vi "Main.vi"() -> ()   [LabVIEW 2020]
uses:
  Def/MHL_Data.ctl
  Def/Queue_Function Def.ctl
  Def/Queue_Method Def.ctl
  Def/Saving Type.ctl
  Def/Watchdog_Data.ctl
  Def/Event Log.ctl
  Objects/Saving Function/Saving OO/Save as csv/Save as csv.lvclass
  D:/Projects/practice/QMH+Producer_consumer/QMH+Producer_consumer/Objects/Saving Function/Saving OO/Saving OO.lvclass
  Def/Queue_Def.ctl
  <userlib>/_MGI/Timing/MGI Wait/MGI Wait (U32).vi
  Objects/Saving Function/Saving OO/Save as txt/Save as txt.lvclass
  Objects/Saving Function/Saving OO/Saving OO.lvclass
panel:
  in  "Connect/Reconnect":bool
  in  "Power":bool
  in  "Decrease Amplitude":bool
  in  "Add Amplitude":bool
  in  "Decrease Frequence":bool
  in  "Increase Frequence":bool
  out "Waveform":dynamicdata(graph)
  in  "MHL Data":T1={"Offset"=0.0, "Frequency"=10.1, "Amplitude"=1.0}
  out "Ver.#":string
  out "error out":errorcluster
  in  "error in (no error)":errorcluster
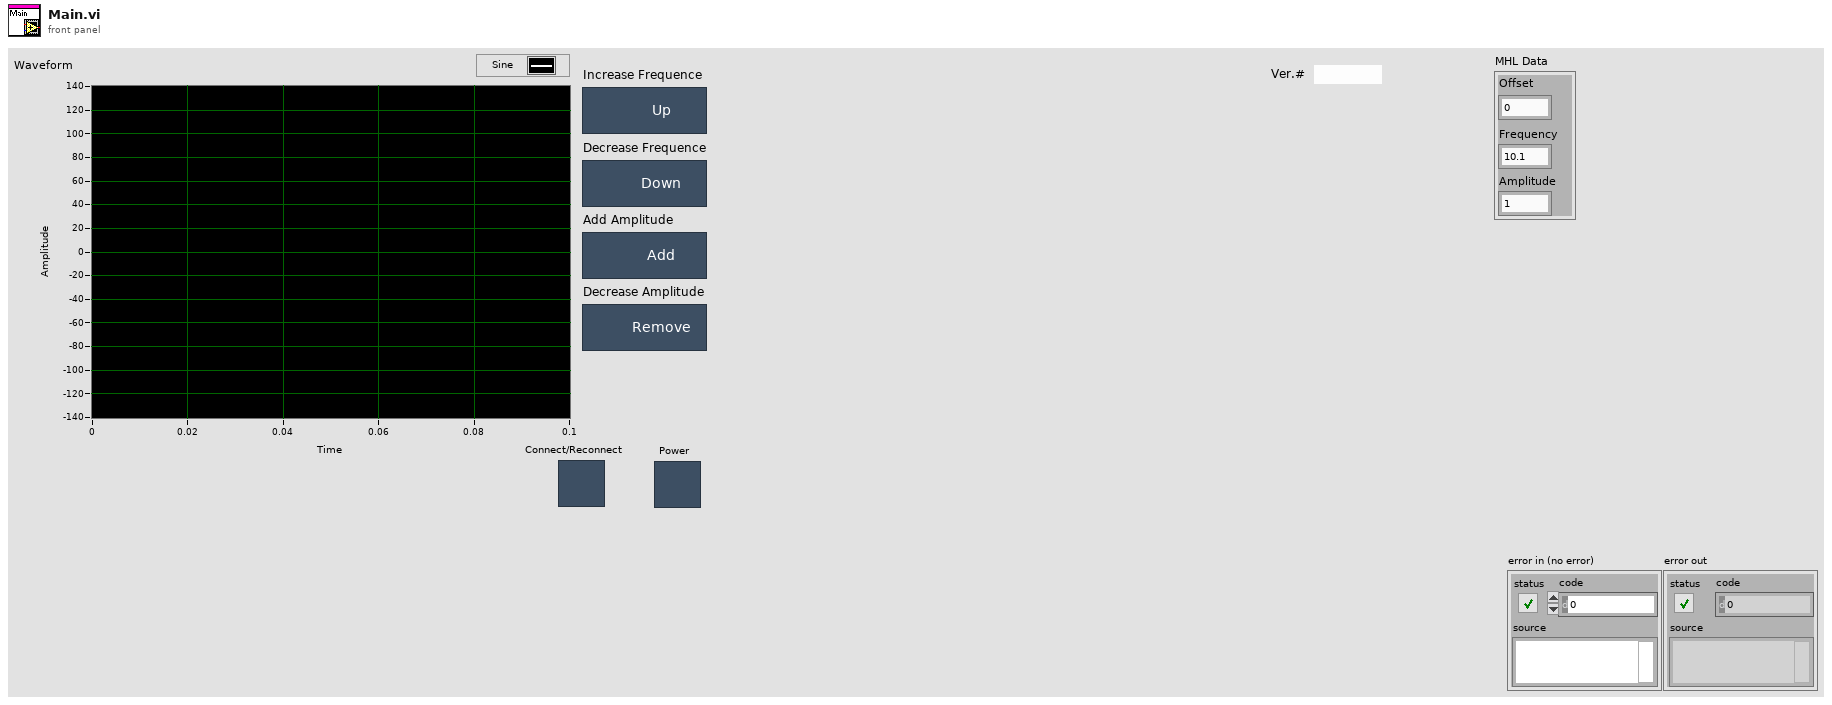
[diagram p1: front panel]
types:
  T1 = typedef "MHL_Data.ctl" = cluster{"Offset":dbl, "Frequency":dbl, "Amplitude":dbl}
  T2 = typedef "Event Log.ctl" = cluster{"Saving Path Folde":path}
  T3 = typedef "Watchdog_Data.ctl" = cluster{string}
  T4 = typedef "Queue_Method Def.ctl" = enum16{"Initialize", "Read", "Write", "Insert", "Get_Specific_Quene_Status", "Flush Speciffic Quene", "Release All Quenes"}
  T5 = typedef "Queue_Function Def.ctl" = enum16{"MHL", "Return(Watch dog)", "Event Log", "Error Log"}
  T6 = typedef "Saving Type.ctl" = enum16{"Default", "txt", "csv"}
  T7 = typedef "Main_Data_Package.ctl" = cluster{"This Vi Ref Out":refnum<vi>, "Map Out":map{string, refnum<vi>}, "User Event Out":refnum<user-event>, "User_Event Ref Reg":refnum<event-registration>, "Event Log Path":path}
  T8 = typedef "Queue_Def.ctl" = cluster{"Message":string, "Data":variant}
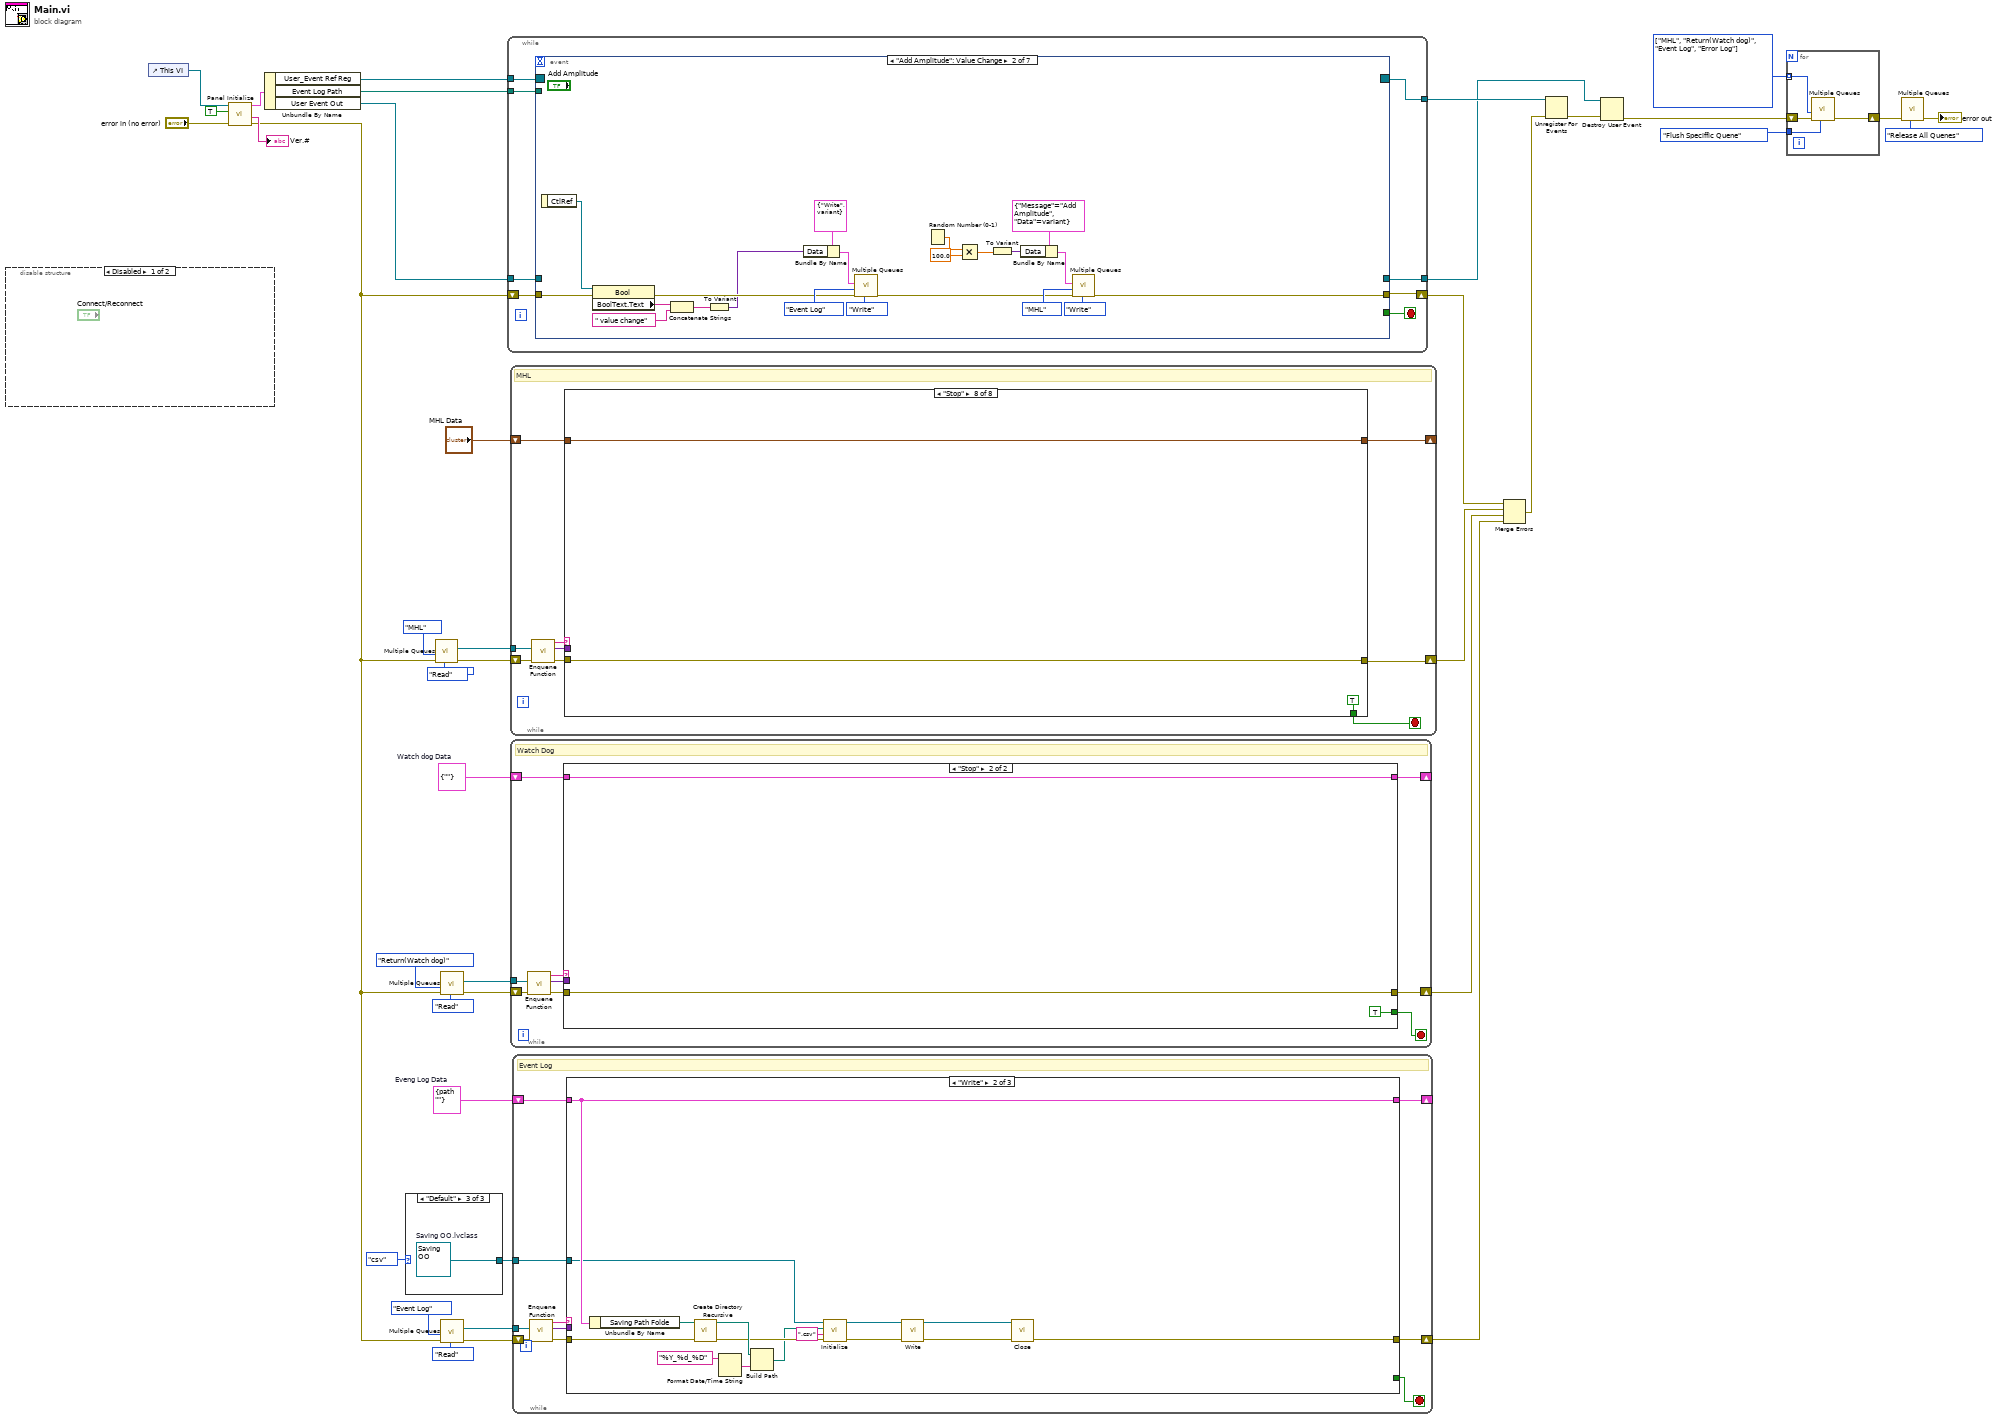
[diagram p0: block diagram]
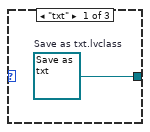
[diagram p3: hidden frame]
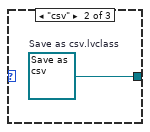
[diagram p4: hidden frame]
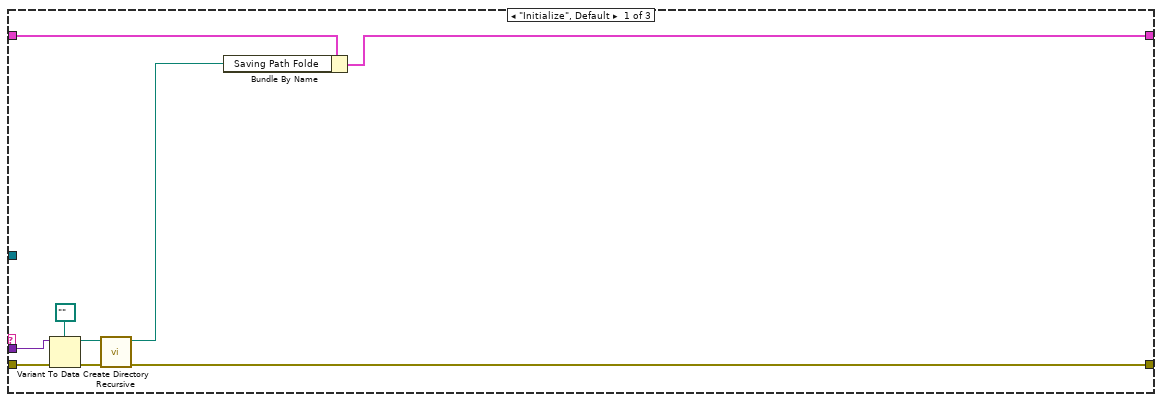
[diagram p5: hidden frame]
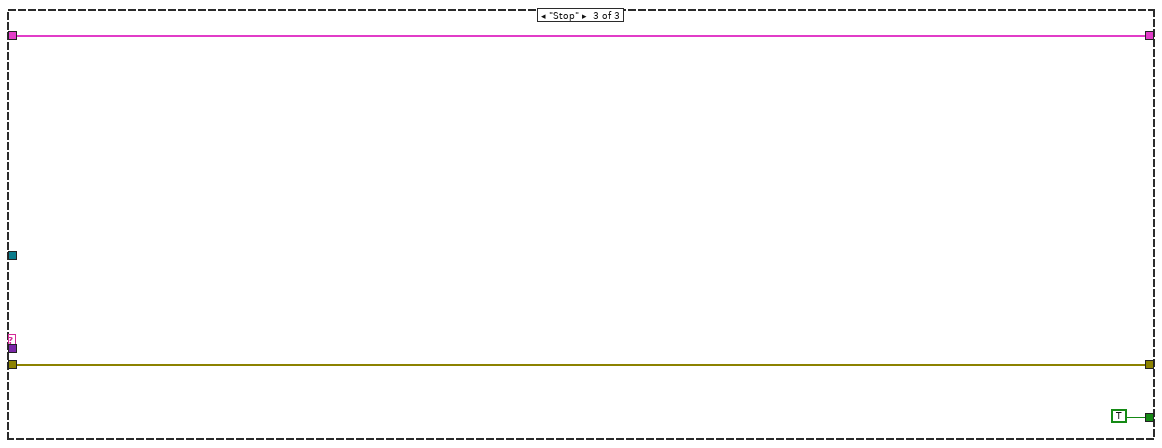
[diagram p6: hidden frame]
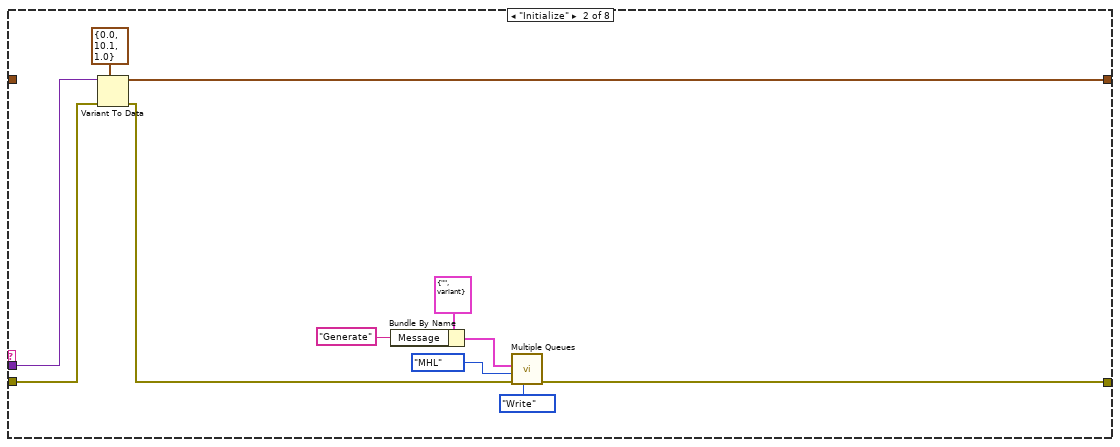
[diagram p9: hidden frame]
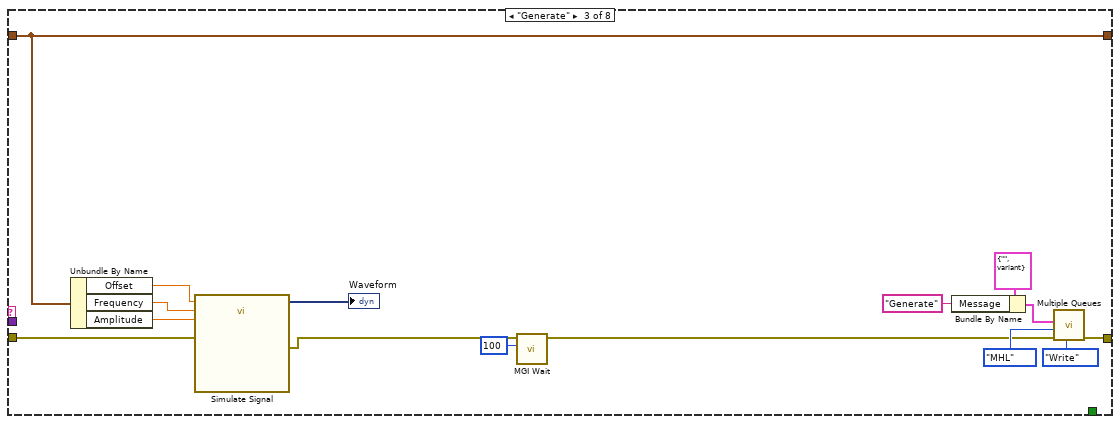
[diagram p10: hidden frame]
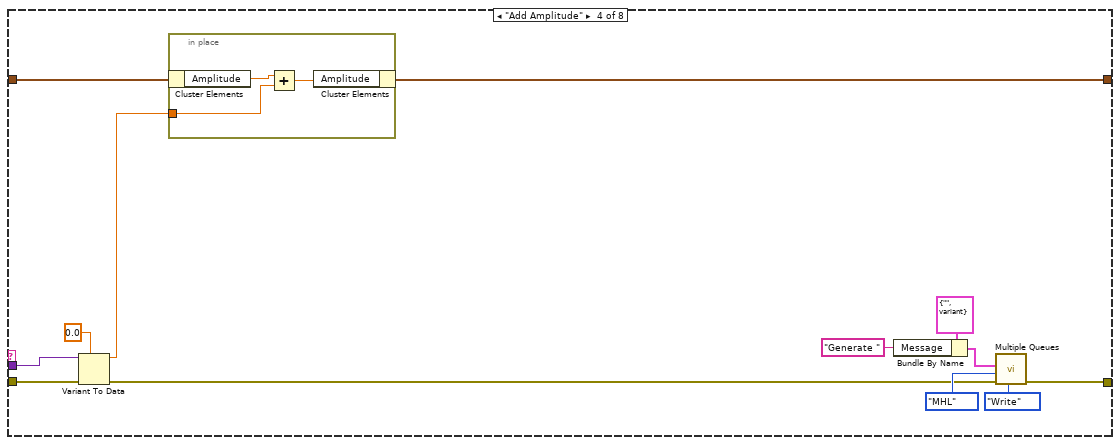
[diagram p11: hidden frame]
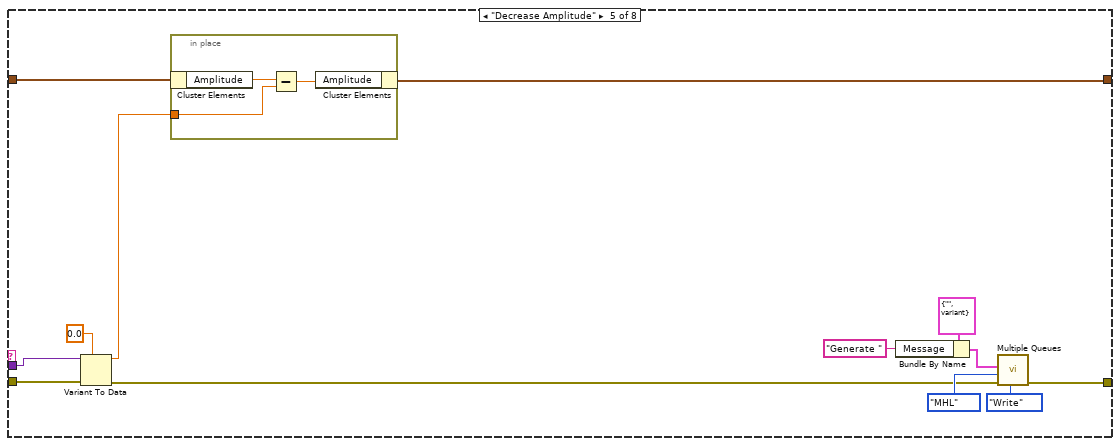
[diagram p12: hidden frame]
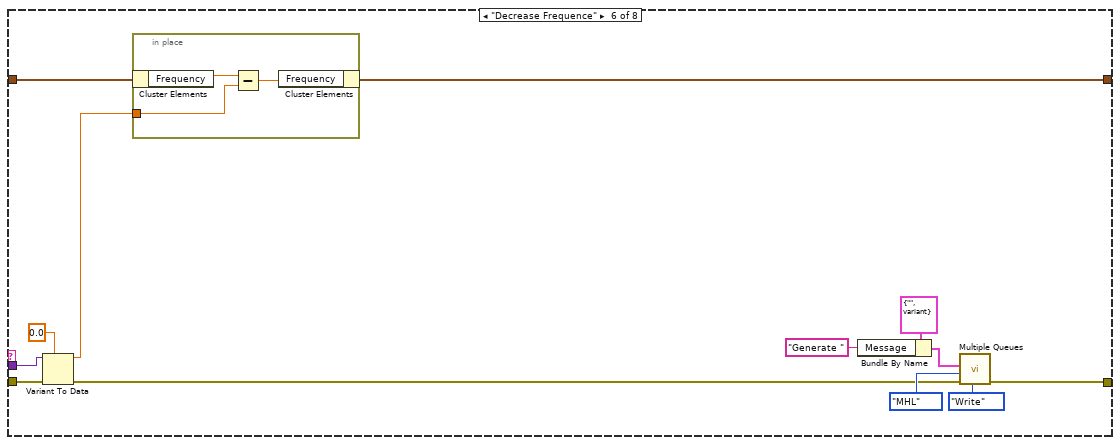
[diagram p13: hidden frame]
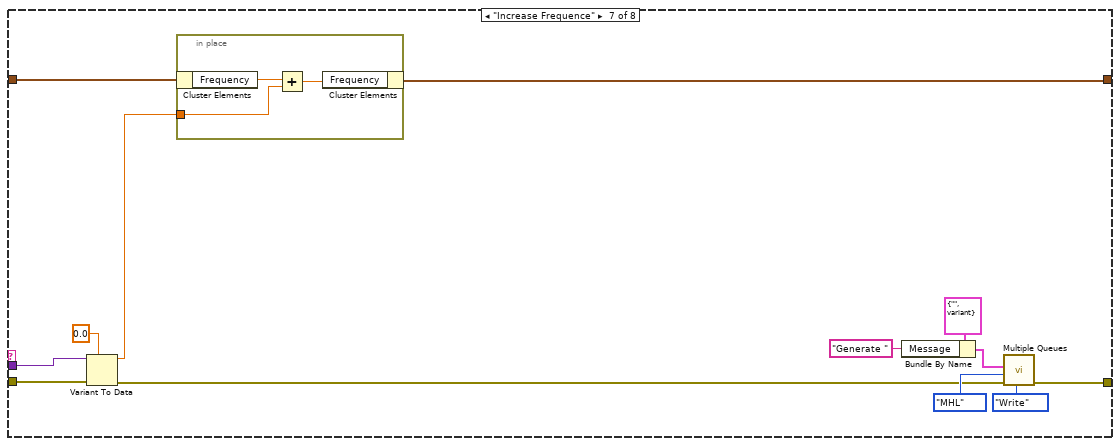
[diagram p14: hidden frame]
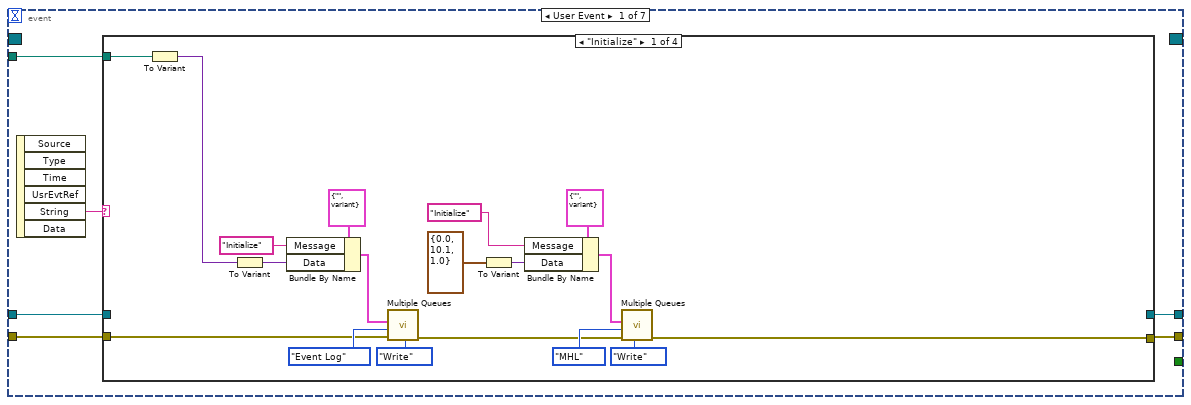
[diagram p15: hidden frame]
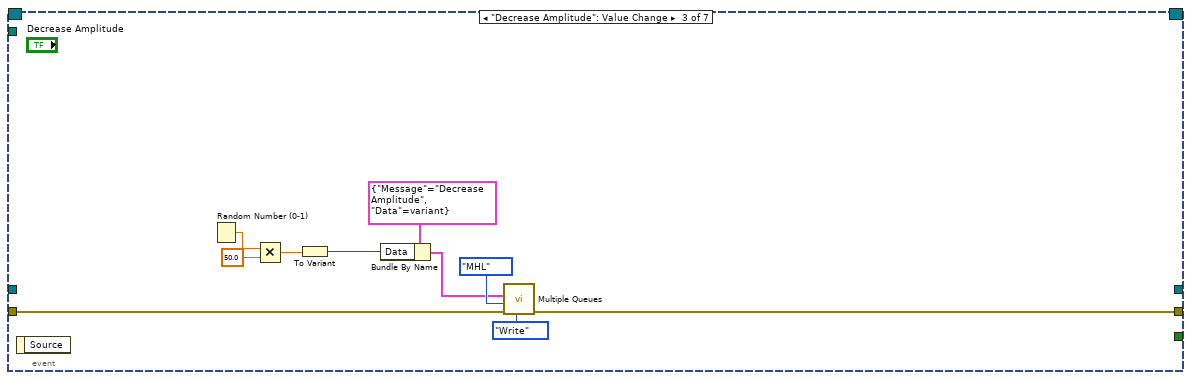
[diagram p19: hidden frame]
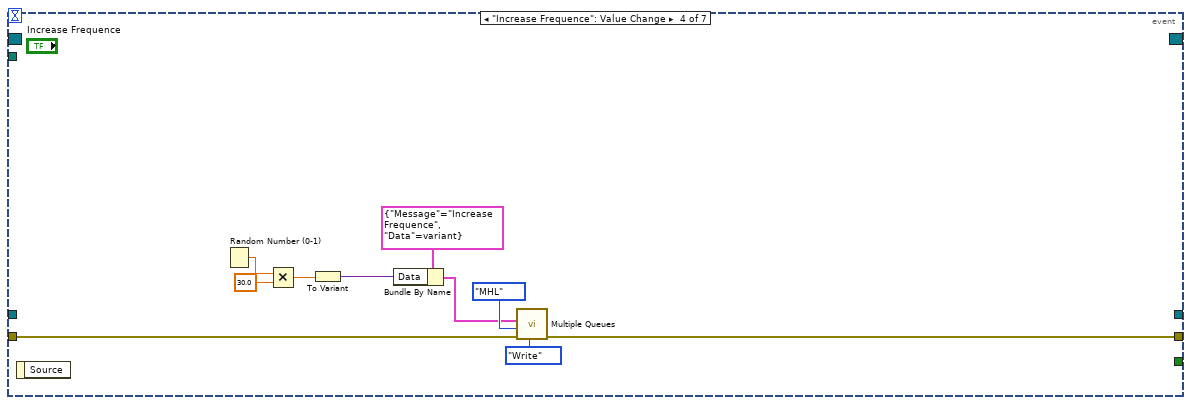
[diagram p20: hidden frame]
diagram:
  w3 = T2 {"Saving Path Folde"=path ""}  # Eveng Log Data
  w4 = T3 {""}  # Watch dog Data
  w31 = T5[] [enum."MHL", enum."Return(Watch dog)", enum."Event Log", enum."Error Log"] items=["MHL", "Return(Watch dog)", "Event Log", "Error Log"]
  n1 = disable-structure shown="Disabled" {
    frame Disabled {
    }
    frame Enabled {
    }
  }
  n2 = control-ref of="This VI"() -> (w40:refnum<vi>)
  n3 = call "Panel Initialize.vi"("error in"="error in (no error)", "Initialize All UI ?"=TRUE, "VI Ref"=w40) -> ("error out"=w7:errorcluster, "Ver.#"=→"Ver.#":string, "Structure Data"=w32:T7)  [unwired: 6 in]
  n4 = Unbundle By Name(w32) -> ("User_Event Ref Reg"=w10:refnum<event-registration>, "Event Log Path"=w1:path, "User Event Out"=w2:refnum<user-event>)
  n5 = case shown="\"Default\"" Saving_Type."csv" ("Saving Type") {
    tunnel: [w41 w42 w43] -> w11
    frame "txt" {
      w41 = refnum<class "Save as txt.lvclass"> refnum  # Save as txt.lvclass
    }
    frame "csv" {
      w42 = refnum<class "Save as csv.lvclass"> refnum  # Save as csv.lvclass
    }
    frame "Default" {
      w43 = refnum<class "Saving OO.lvclass"> refnum  # Saving OO.lvclass
    }
  }
  n6 = call "Multiple Queues.vi"("Method"=Queue_Method_Def."Read", "error in"=w7, "Functions"=Queue_Function_Def."MHL") -> ("error out"=w5:errorcluster, "queue out"=w6:refnum<queue>)  [unwired: 6 in, 1 out]
  n7 = call "Multiple Queues.vi"("Method"=Queue_Method_Def."Read", "error in"=w7, "Functions"=Queue_Function_Def."Return(Watch dog)") -> ("error out"=w21:errorcluster, "queue out"=w20:refnum<queue>)  [unwired: 6 in, 1 out]
  n8 = call "Multiple Queues.vi"("Method"=Queue_Method_Def."Read", "error in"=w7, "Functions"=Queue_Function_Def."Event Log") -> ("error out"=w14:errorcluster, "queue out"=w15:refnum<queue>)  [unwired: 6 in, 1 out]
  n9 = while {
    tunnel: w10 -> [w50]
    tunnel: [w49] -> w37
    shift-right: [w46] -> w36
    shift-left: w7 -> [w48]
    tunnel: w2 -> [w47]
    tunnel: [w45] -> w33
    tunnel: w1 -> [w44]
    stop <- w51 stop-if-true
    n10 = event shown="[1] \"Add Amplitude\": Value Change" {
      selector: w50 -> [_ _ _ _ _ _ _]
      dyn-events: [_ _ _ _ _ _ _] -> w49
      timeout: _ -> [_ _ _ _ _ _ _]
      tunnel: [_ _ _ _ _ TRUE ("Discard?") w144] -> w51
      tunnel: w48 -> [w57 w86 w103 w113 w123 w134 w143]
      tunnel: w47 -> [w56 _ _ _ _ _ _]
      tunnel: [w55 w88 w102 w112 w122 w133 w142] -> w46
      tunnel: [w54 _ _ _ _ _ _] -> w45
      tunnel: w44 -> [w52 _ _ _ _ _ _]
      event User Event {
        n11 = event-data() -> ("String"=w53:string)  [unwired: 1 in, 5 out]
        n12 = case shown="\"Initialize\"" w53 {
          tunnel: w57 -> [w62 w77 w78 w80]
          tunnel: w56 -> [_ w76 w79 _]
          tunnel: [w60 w77 w78 w80] -> w55
          tunnel: [_ w76 w79 _] -> w54
          tunnel: w52 -> [w63 _ _ _]
          frame "Initialize" {
            n13 = To Variant(anything=w63) -> (Variant=w58:variant)
            n14 = To Variant(anything=w58) -> (Variant=w59:variant)
            n15 = Bundle By Name(cluster=T8 {"Message"="", "Data"=variant} ("Quenes"), "Message"="Initialize", "Data"=w59) -> (w64:T8)
            n16 = call "Multiple Queues.vi"("Method"=Queue_Method_Def."Write", "error in"=w62, "Functions"=Queue_Function_Def."Event Log", "Quenes"=w64) -> ("error out"=w61:errorcluster)  [unwired: 5 in, 2 out]
            n17 = To Variant(anything=T1 {"Offset"=0.0, "Frequency"=10.1, "Amplitude"=1.0} ("MHL Data")) -> (Variant=w71:variant)
            n18 = Bundle By Name(cluster=T8 {"Message"="", "Data"=variant} ("Quenes"), "Message"="Initialize", "Data"=w71) -> (w69:T8)
            n19 = call "Multiple Queues.vi"("Method"=Queue_Method_Def."Write", "error in"=w61, "Functions"=Queue_Function_Def."MHL", "Quenes"=w69) -> ("error out"=w60:errorcluster)  [unwired: 5 in, 2 out]
          }
          frame "Write a Log" {
          }
          frame "Refresh" {
          }
          frame Default {
          }
        }
      }
      event "Add Amplitude": Value Change {
        n20 = event-data() -> ("CtlRef"=w85:refnum<vi>)  [unwired: 1 in]
        n21 = property class="Bool"(reference=w85, error in=w86) -> (error out=w87:errorcluster, "BoolText.Text"=w84:string)  [unwired: 1 out]
        n22 = Concatenate Strings(w84, " value change") -> (w82:string)
        n23 = To Variant(anything=w82) -> (Variant=w81:variant)
        n24 = Bundle By Name(cluster=T8 {"Message"="Write", "Data"=variant} ("Quenes"), "Data"=w81) -> (w93:T8)
        n25 = call "Multiple Queues.vi"("Method"=Queue_Method_Def."Write", "error in"=w87, "Functions"=Queue_Function_Def."Event Log", "Quenes"=w93) -> ("error out"=w89:errorcluster)  [unwired: 5 in, 2 out]
        n26 = Random Number (0-1)() -> (number: 0 to 1=w98:dbl)
        n27 = Multiply(x=w98, y=100.0) -> (x*y=w96:dbl)
        n28 = To Variant(anything=w96) -> (Variant=w95:variant)
        n29 = Bundle By Name(cluster=T8 {"Message"="Add Amplitude", "Data"=variant} ("Quenes"), "Data"=w95) -> (w94:T8)
        n30 = call "Multiple Queues.vi"("Method"=Queue_Method_Def."Write", "error in"=w89, "Functions"=Queue_Function_Def."MHL", "Quenes"=w94) -> ("error out"=w88:errorcluster)  [unwired: 5 in, 2 out]
      }
      event "Decrease Amplitude": Value Change {
        n31 = event-data() -> ()  [unwired: 1 in, 1 out]
        n32 = Random Number (0-1)() -> (number: 0 to 1=w108:dbl)
        n33 = Multiply(x=w108, y=50.0) -> (x*y=w106:dbl)
        n34 = To Variant(anything=w106) -> (Variant=w105:variant)
        n35 = Bundle By Name(cluster=T8 {"Message"="Decrease Amplitude", "Data"=variant} ("Quenes"), "Data"=w105) -> (w104:T8)
        n36 = call "Multiple Queues.vi"("Method"=Queue_Method_Def."Write", "error in"=w103, "Functions"=Queue_Function_Def."MHL", "Quenes"=w104) -> ("error out"=w102:errorcluster)  [unwired: 5 in, 2 out]
      }
      event "Increase Frequence": Value Change {
        n37 = event-data() -> ()  [unwired: 1 in, 1 out]
        n38 = Random Number (0-1)() -> (number: 0 to 1=w118:dbl)
        n39 = Multiply(x=w118, y=30.0) -> (x*y=w116:dbl)
        n40 = To Variant(anything=w116) -> (Variant=w115:variant)
        n41 = Bundle By Name(cluster=T8 {"Message"="Increase Frequence", "Data"=variant} ("Quenes"), "Data"=w115) -> (w114:T8)
        n42 = call "Multiple Queues.vi"("Method"=Queue_Method_Def."Write", "error in"=w113, "Functions"=Queue_Function_Def."MHL", "Quenes"=w114) -> ("error out"=w112:errorcluster)  [unwired: 5 in, 2 out]
      }
      event "Decrease Frequence": Value Change {
        n43 = event-data() -> ()  [unwired: 1 in, 1 out]
        n44 = Random Number (0-1)() -> (number: 0 to 1=w128:dbl)
        n45 = Multiply(x=w128, y=15.0) -> (x*y=w126:dbl)
        n46 = To Variant(anything=w126) -> (Variant=w125:variant)
        n47 = Bundle By Name(cluster=T8 {"Message"="Decrease Frequence", "Data"=variant} ("Quenes"), "Data"=w125) -> (w124:T8)
        n48 = call "Multiple Queues.vi"("Method"=Queue_Method_Def."Write", "error in"=w123, "Functions"=Queue_Function_Def."MHL", "Quenes"=w124) -> ("error out"=w122:errorcluster)  [unwired: 5 in, 2 out]
      }
      event "Power": Value Change {
        w135 = T5[] [enum."MHL", enum."Return(Watch dog)", enum."Event Log", enum."Error Log"] items=["MHL", "Return(Watch dog)", "Event Log", "Error Log"]
        n49 = event-data() -> ()  [unwired: 1 in, 1 out]
        n50 = for {
          tunnel: w135 -> [w137] mode=indexing
          tunnel: w134 -> [w140]
          tunnel: [w139] -> w133
          n51 = call "Multiple Queues.vi"("Method"=Queue_Method_Def."Insert", "error in"=w140, "Functions"=w137, "Quenes"=T8 {"Message"="Stop", "Data"=variant}) -> ("error out"=w139:errorcluster)  [unwired: 5 in, 2 out]
        }
      }
      event Panel Close? {
        w141 = T5[] [enum."MHL", enum."Return(Watch dog)", enum."Event Log", enum."Error Log"] items=["MHL", "Return(Watch dog)", "Event Log", "Error Log"]
        w144 = TRUE ("Discard?")
        n52 = event-data() -> ()  [unwired: 1 in, 1 out]
        n53 = for {
          tunnel: w141 -> [w146] mode=indexing
          tunnel: w143 -> [w149]
          tunnel: [w148] -> w142
          n54 = call "Multiple Queues.vi"("Method"=Queue_Method_Def."Insert", "error in"=w149, "Functions"=w146, "Quenes"=T8 {"Message"="Stop", "Data"=variant}) -> ("error out"=w148:errorcluster)  [unwired: 5 in, 2 out]
        }
        n55 = event-data("Discard?"=w144) -> ()  [unwired: 1 in, 1 out]
      }
    }
  }
  n56 = while {
    shift-right: [w157] -> w35
    shift-left: w5 -> [w151]
    shift-right: [w153] -> _
    shift-left: "MHL Data" -> [w150]
    tunnel: w6 -> [w152]
    stop <- w158 stop-if-true
    # "MHL"
    n57 = call "Enquene Function.vi"("error in (no error)"=w151, "Queue"=w152) -> ("error out"=w156:errorcluster, "Data"=w154:variant, "Message"=w155:string)  [unwired: 7 in]
    n58 = case shown="\"Stop\"" w155 {
      tunnel: [_ _ _ _ _ _ _ TRUE] -> w158
      tunnel: [w160 w166 w182 w189 w205 w220 w235 w252] -> w157
      tunnel: w156 -> [w160 w168 w186 w199 w207 w222 w239 w252]
      tunnel: w154 -> [_ w170 _ w198 w206 w221 w238 _]
      tunnel: [w159 w167 w175 w187 w203 w219 w236 w251] -> w153
      tunnel: w150 -> [w159 _ w175 w188 w204 w223 w237 w251]
      frame Default {
      }
      frame "Initialize" {
        n59 = Variant To Data(error in=w168, type=T1 {"Offset"=0.0, "Frequency"=10.1, "Amplitude"=1.0} ("MHL Data"), Variant=w170) -> (data=w167:T1, error out=w169:errorcluster)
        n60 = Bundle By Name(cluster=T8 {"Message"="", "Data"=variant} ("Quenes"), "Message"="Generate") -> (w162:T8)
        n61 = call "Multiple Queues.vi"("Method"=Queue_Method_Def."Write", "error in"=w169, "Functions"=Queue_Function_Def."MHL", "Quenes"=w162) -> ("error out"=w166:errorcluster)  [unwired: 5 in, 2 out]
      }
      frame "Generate" {
        n62 = Unbundle By Name(w175) -> ("Offset"=w174:dbl, "Frequency"=w173:dbl, "Amplitude"=w172:dbl)
        n63 = call "Simulate Signal"("Offset"=w174, "Frequency"=w173, "Amplitude"=w172, "error in (no error)"=w186) -> ("Sine"=→"Waveform":dynamicdata, "error out"=w183:errorcluster)  [unwired: 10 in]
        n64 = call-poly <userlib>:"MGI Wait.vi"("ms"=u32 100, "Error In"=w183) -> ("Error Out"=w178:errorcluster)  [unwired: 5 in]
        n65 = Bundle By Name(cluster=T8 {"Message"="", "Data"=variant} ("Quenes"), "Message"="Generate") -> (w179:T8)
        n66 = call "Multiple Queues.vi"("Method"=Queue_Method_Def."Write", "error in"=w178, "Functions"=Queue_Function_Def."MHL", "Quenes"=w179) -> ("error out"=w182:errorcluster)  [unwired: 5 in, 2 out]
      }
      frame "Add Amplitude" {
        n67 = Variant To Data(error in=w199, type=0.0, Variant=w198) -> (data=w196:dbl, error out=w190:errorcluster)
        n68 = in-place {
          in-place-border: w196 -> [w202]
          n69 = in-place-cluster #1(w188) -> ("Amplitude"=w200:dbl)
          n70 = Add(x=w200, y=w202) -> (x+y=w201:dbl)
          n71 = in-place-cluster #1("Amplitude"=w201) -> (w187:T1)
        }
        n72 = Bundle By Name(cluster=T8 {"Message"="", "Data"=variant} ("Quenes"), "Message"="Generate ") -> (w191:T8)
        n73 = call "Multiple Queues.vi"("Method"=Queue_Method_Def."Write", "error in"=w190, "Functions"=Queue_Function_Def."MHL", "Quenes"=w191) -> ("error out"=w189:errorcluster)  [unwired: 5 in, 2 out]
      }
      frame "Decrease Amplitude" {
        n74 = Variant To Data(error in=w207, type=0.0, Variant=w206) -> (data=w214:dbl, error out=w208:errorcluster)
        n75 = in-place {
          in-place-border: w214 -> [w218]
          n76 = in-place-cluster #2(w204) -> ("Amplitude"=w216:dbl)
          n77 = Subtract(x=w216, y=w218) -> (x-y=w217:dbl)
          n78 = in-place-cluster #2("Amplitude"=w217) -> (w203:T1)
        }
        n79 = Bundle By Name(cluster=T8 {"Message"="", "Data"=variant} ("Quenes"), "Message"="Generate ") -> (w209:T8)
        n80 = call "Multiple Queues.vi"("Method"=Queue_Method_Def."Write", "error in"=w208, "Functions"=Queue_Function_Def."MHL", "Quenes"=w209) -> ("error out"=w205:errorcluster)  [unwired: 5 in, 2 out]
      }
      frame "Decrease Frequence" {
        n81 = Variant To Data(error in=w222, type=0.0, Variant=w221) -> (data=w230:dbl, error out=w224:errorcluster)
        n82 = in-place {
          in-place-border: w230 -> [w234]
          n83 = in-place-cluster #3(w223) -> ("Frequency"=w232:dbl)
          n84 = Subtract(x=w232, y=w234) -> (x-y=w233:dbl)
          n85 = in-place-cluster #3("Frequency"=w233) -> (w219:T1)
        }
        n86 = Bundle By Name(cluster=T8 {"Message"="", "Data"=variant} ("Quenes"), "Message"="Generate ") -> (w225:T8)
        n87 = call "Multiple Queues.vi"("Method"=Queue_Method_Def."Write", "error in"=w224, "Functions"=Queue_Function_Def."MHL", "Quenes"=w225) -> ("error out"=w220:errorcluster)  [unwired: 5 in, 2 out]
      }
      frame "Increase Frequence" {
        n88 = Variant To Data(error in=w239, type=0.0, Variant=w238) -> (data=w246:dbl, error out=w240:errorcluster)
        n89 = in-place {
          in-place-border: w246 -> [w250]
          n90 = in-place-cluster #4(w237) -> ("Frequency"=w248:dbl)
          n91 = Add(x=w248, y=w250) -> (x+y=w249:dbl)
          n92 = in-place-cluster #4("Frequency"=w249) -> (w236:T1)
        }
        n93 = Bundle By Name(cluster=T8 {"Message"="", "Data"=variant} ("Quenes"), "Message"="Generate ") -> (w241:T8)
        n94 = call "Multiple Queues.vi"("Method"=Queue_Method_Def."Write", "error in"=w240, "Functions"=Queue_Function_Def."MHL", "Quenes"=w241) -> ("error out"=w235:errorcluster)  [unwired: 5 in, 2 out]
      }
      frame "Stop" {
      }
    }
  }
  n95 = while {
    tunnel: w20 -> [w256]
    shift-right: [w260] -> w19
    shift-left: w21 -> [w262]
    shift-right: [w254] -> _
    shift-left: w4 -> [w255]
    stop <- w257 stop-if-true
    # "Watch Dog"
    n96 = call "Enquene Function.vi"("error in (no error)"=w262, "Queue"=w256) -> ("error out"=w261:errorcluster, "Data"=w258:variant, "Message"=w259:string)  [unwired: 7 in]
    n97 = case shown="\"Stop\"" w259 {
      tunnel: [w264 w267] -> w260
      tunnel: w261 -> [w264 w267]
      tunnel: w258 -> [_ _]
      tunnel: [_ TRUE] -> w257
      tunnel: w255 -> [w263 w265]
      tunnel: [w263 w265] -> w254
      frame "False", Default {
      }
      frame "Stop" {
      }
    }
  }
  n98 = while {
    shift-right: [w275] -> w13
    shift-left: w14 -> [w277]
    tunnel: w15 -> [w270]
    tunnel: w11 -> [w271]
    shift-right: [w268] -> _
    shift-left: w3 -> [w269]
    stop <- w272 stop-if-true
    # "Event Log"
    n99 = call "Enquene Function.vi"("error in (no error)"=w277, "Queue"=w270) -> ("error out"=w276:errorcluster, "Data"=w273:variant, "Message"=w274:string)  [unwired: 7 in]
    n100 = case shown="\"Write\"" w274 {
      tunnel: [w279 w292 w303] -> w275
      tunnel: w276 -> [w283 w294 w303]
      tunnel: w273 -> [w282 _ _]
      tunnel: [_ _ TRUE] -> w272
      tunnel: w271 -> [_ w288 _]
      tunnel: w269 -> [w280 w291 w302]
      tunnel: [w281 w291 w302] -> w268
      frame "Initialize", Default {
        n101 = Variant To Data(error in=w283, type=path "", Variant=w282) -> (data=w285:path, error out=w284:errorcluster)
        n102 = call <vilib>:"Create Directory Recursive.vi"("error in (no error)"=w284, "directory"=w285) -> ("error out"=w279:errorcluster, "directory copy"=w278:path)  [unwired: 3 in, 1 out]
        n103 = Bundle By Name(cluster=w280, "Saving Path Folde"=w278) -> (w281:T2)
      }
      frame "Write" {
        n104 = Unbundle By Name(w291) -> ("Saving Path Folde"=w289:path)
        n105 = call <vilib>:"Create Directory Recursive.vi"("error in (no error)"=w294, "directory"=w289) -> ("error out"=w293:errorcluster, "directory copy"=w299:path)  [unwired: 3 in, 1 out]
        n106 = Format Date/Time String(time format string (%c)="%Y_%d_%D") -> (date/time string=w300:string)  [unwired: 2 in]
        n107 = Build Path(base path=w299, name or relative path=w300) -> (appended path=w290:path)
        n108 = call-dynamic "Initialize.vi"("error in (no error)"=w293, "type"=".csv", "Path"=w290, "Saving OO in"=w288) -> ("error out"=w296:errorcluster, "Saving OO out"=w298:refnum<class "Saving OO.lvclass">)  [unwired: 6 in]
        n109 = call-dynamic "Write.vi"("error in (no error)"=w296, "Saving OO in"=w298) -> ("error out"=w295:errorcluster, "Saving OO out"=w297:refnum<class "Saving OO.lvclass">)  [unwired: 8 in]
        n110 = call-dynamic "Close.vi"("error in (no error)"=w295, "Saving OO in"=w297) -> ("error out"=w292:errorcluster)  [unwired: 8 in, 1 out]
      }
      frame "Stop" {
      }
    }
  }
  n111 = Merge Errors(w36, w35, w19, w13) -> (w34:errorcluster)
  n112 = Unregister For Events(event registration refnum=w37, error in=w34) -> (error out=w38:errorcluster)
  n113 = Destroy User Event(user event=w33, error in=w38) -> (error out=w30:errorcluster)
  n114 = for {
    tunnel: w31 -> [w308] mode=indexing
    shift-right: [w306] -> w29
    shift-left: w30 -> [w307]
    tunnel: Queue_Method_Def."Flush Speciffic Quene" ("Method") -> [w305]
    n115 = call "Multiple Queues.vi"("Method"=w305, "error in"=w307, "Functions"=w308) -> ("error out"=w306:errorcluster)  [unwired: 6 in, 2 out]
  }
  n116 = call "Multiple Queues.vi"("Method"=Queue_Method_Def."Release All Quenes", "error in"=w29) -> ("error out"=→"error out":errorcluster)  [unwired: 7 in, 2 out]
